vi "TX focus FOCO.vi"(0 "Comando":string, 9 "Setpoint":dbl min=0.0 max=360.0) -> (4 "pos (deg)":dbl min=0.0 max=360.0 format="%.2f", 10 "Parou":bool, 15 "mec position":dbl min=0.0 max=360.0 format="%.2f")   [LabVIEW 2012]
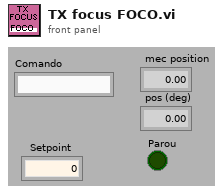
[diagram p1: front panel]
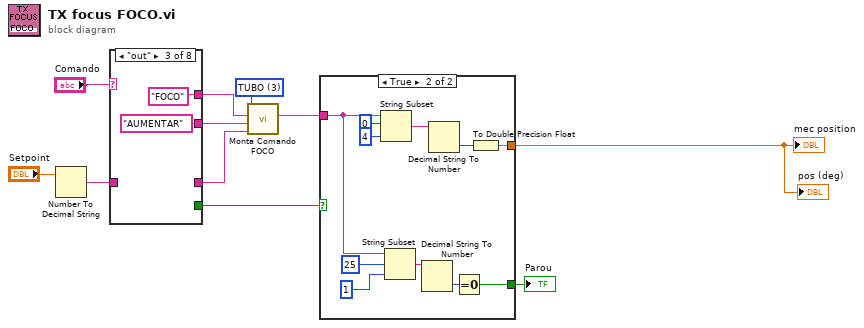
[diagram p0: block diagram]
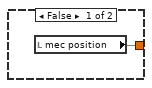
[diagram p2: hidden frame]
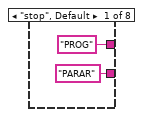
[diagram p3: hidden frame]
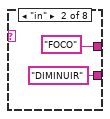
[diagram p4: hidden frame]
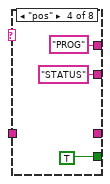
[diagram p5: hidden frame]
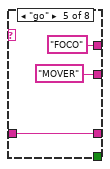
[diagram p6: hidden frame]
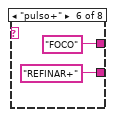
[diagram p7: hidden frame]
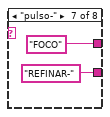
[diagram p8: hidden frame]
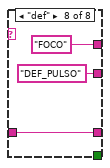
[diagram p9: hidden frame]
diagram:
  w2 = u16 3 items=["ZERO", "AH", "DEC", "TUBO", "CUP"] ("Controlador")
  n1 = Number To Decimal String(number="Setpoint") -> (decimal integer string=w9:string)  [unwired: 1 in]
  n2 = case shown="\"out\"" "Comando" {
    tunnel: w9 -> [_ _ _ _ w22 _ _ w28]
    tunnel: ["PARAR" ("Comando") "DIMINUIR" ("Comando") "AUMENTAR" ("Comando") "STATUS" ("Comando") "MOVER" ("Comando") "REFINAR+" ("Comando") "REFINAR-" ("Comando") "DEF_PULSO" ("Comando")] -> w4
    tunnel: [_ _ _ _ w22 _ _ w28] -> w3
    tunnel: [_ _ _ TRUE _ _ _ _] -> w8
    tunnel: ["PROG" ("Comando") "FOCO" ("Comando") "FOCO" ("Comando") "PROG" ("Comando") "FOCO" ("Comando") "FOCO" ("Comando") "FOCO" ("Comando") "FOCO" ("Comando")] -> w5
    frame "stop", Default {
    }
    frame "in" {
    }
    frame "out" {
    }
    frame "pos" {
    }
    frame "go" {
    }
    frame "pulso+" {
    }
    frame "pulso-" {
    }
    frame "def" {
    }
  }
  n3 = call "Monta Comando FOCO.vi"("Set Point"=w3, "Comando"=w4, "Dispositivo"=w5, "Controlador"=w2) -> ("Resposta"=w6:string)  [unwired: 3 in, 2 out]
  n4 = case shown="True" w8 {
    tunnel: w6 -> [_ w32]
    tunnel: [w31 w39] -> w1
    tunnel: [_ w33] -> w7
    frame False {
      n5 = local read "mec position"() -> (w31:dbl)
    }
    frame True {
      n6 = String Subset(string=w32, offset (0)=0, length (rest)=4 ("length (rest)")) -> (substring=w41:string)
      n7 = String Subset(string=w32, offset (0)=25, length (rest)=1 ("length (rest)")) -> (substring=w35:string)
      n8 = Decimal String To Number(string=w35) -> (number=w34:i32)  [unwired: 2 in, 1 out]
      n9 = Decimal String To Number(string=w41) -> (number=w40:i32)  [unwired: 2 in, 1 out]
      n10 = Equal To 0?(x=w34) -> (x = 0?=w33:bool)
      n11 = To Double Precision Float(number=w40) -> (double precision float=w39:dbl)
    }
  }
  "pos (deg)" <- w1
  "mec position" <- w1
  "Parou" <- w7
